vi "NI-SWITCH Initialize Simulated Session.vi"(8 "error in (no error)":errorcluster, 11 "topology":string) -> (0 "error out":errorcluster, 3 "NI-SWITCH session":refnum<k15>)   [LabVIEW 2017, in "NI-SWITCH Messaging.lvlib" / "NI-SWITCH Consumer.lvclass"]
uses:
  NI-SWITCH Consumer.lvclass
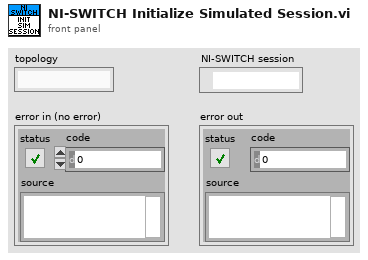
[diagram p1: front panel]
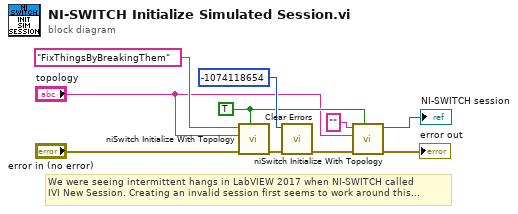
[diagram p0: block diagram]
diagram:
  w5 = TRUE ("simulate (boolean value)")
  # "We were seeing intermittent hangs in LabVIEW 2017 when NI-SWITCH called\nIVI New Session. Creating an invalid session first seems to work around this..."
  n1 = call <instrlib>:"niSwitch Initialize With Topology.vi"("simulate (boolean value)"=w5, "error in (no error)"="error in (no error)", "topology name"="topology", "resource name"="FixThingsByBreakingThem") -> ("error out"=w7:errorcluster)  [unwired: 6 in, 1 out]
  n2 = call <vilib>:"Clear Errors.vi"("error in (no error)"=w7, "specific error code to clear (0: all)"=-1074118654) -> ("error out"=w6:errorcluster)  [unwired: 4 in, 1 out]
  n3 = call <instrlib>:"niSwitch Initialize With Topology.vi"("simulate (boolean value)"=w5, "error in (no error)"=w6, "topology name"="topology", "resource name"="") -> ("error out"=→"error out":errorcluster, "instrument handle out"=→"NI-SWITCH session":refnum<k15>)  [unwired: 6 in]
